vi "Fail If.vi"(7 "Description":string, 8 "error in (no error)":errorcluster, 9 "Message":string, 10 "Fail?":bool, 11 "LUnit Test Case In":refnum<class "LUnit Test Case.lvclass">) -> (0 "error out":errorcluster, 3 "LUnit Test Case Out":refnum<class "LUnit Test Case.lvclass">)   [LabVIEW 2020, in "LUnit Test Case.lvclass"]
doc: "Generates a fail result for the calling test method if the conditional input is true. A description and message may be provided."
uses:
  LUnit Test Case.lvclass
  Result Classes/Assertion Result/Public/TypeDefs/Assertion Type.ctl
  Result Classes/Assertion Result/Assertion Result.lvclass
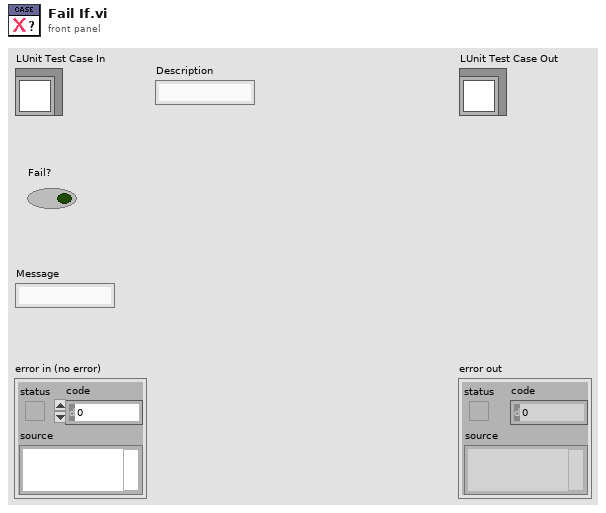
[diagram p1: front panel]
types:
  T1 = typedef "Assertion Result.lvclass/Assertion Type.ctl" = enum16{"None", "Pass", "Fail", "Skip", "Pass if Equal", "Fail if Equal", "Pass if Error", "Fail if Error", "Pass if", "Fail if"}
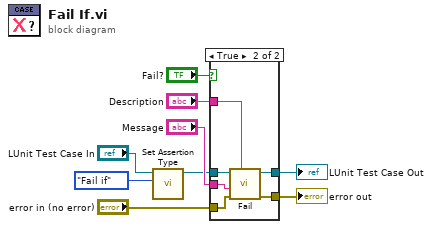
[diagram p0: block diagram]
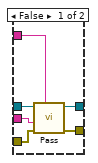
[diagram p2: hidden frame]
diagram:
  n1 = call "Set Assertion Type.vi"("Assertion Type"=Assertion_Type."Fail if", "LUnit Test Case In"="LUnit Test Case In") -> ("LUnit Test Case Out"=w3:refnum<class "LUnit Test Case.lvclass">)  [unwired: 9 in]
  n2 = case shown="True" "Fail?" {
    tunnel: [w15 w20] -> w8
    tunnel: [w11 w19] -> w4
    tunnel: "Description" -> [w13 w17]
    tunnel: "Message" -> [w12 w18]
    tunnel: w3 -> [w14 w21]
    tunnel: "error in (no error)" -> [w10 w16]
    frame False {
      n3 = call "Pass.vi"("Description"=w13, "error in (no error)"=w10, "Message"=w12, "LUnit Test Case In"=w14) -> ("error out"=w11:errorcluster, "LUnit Test Case Out"=w15:refnum<class "LUnit Test Case.lvclass">)  [unwired: 6 in]
    }
    frame True {
      n4 = call "Fail.vi"("Description"=w17, "error in (no error)"=w16, "Message"=w18, "LUnit Test Case In"=w21) -> ("error out"=w19:errorcluster, "LUnit Test Case Out"=w20:refnum<class "LUnit Test Case.lvclass">)  [unwired: 6 in]
    }
  }
  "error out" <- w4
  "LUnit Test Case Out" <- w8
